vi "headers.vi"(8 "error in (no error)":errorcluster, 10 "string":string, 11 "Byte Stream File in":refnum<file>) -> (0 "error out":errorcluster, 3 "Byte Stream File out":refnum<file>)   [LabVIEW 2019]
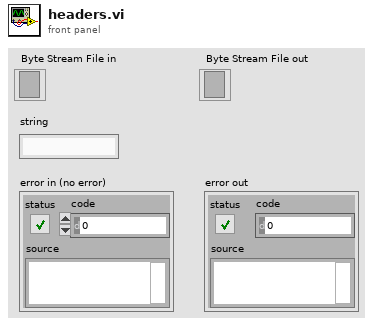
[diagram p1: front panel]
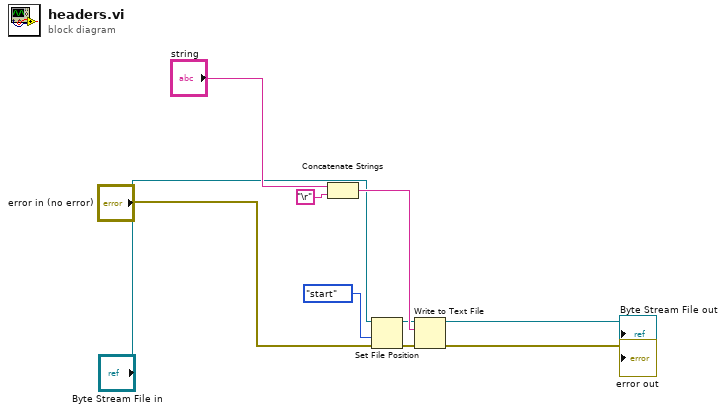
[diagram p0: block diagram]
diagram:
  n1 = Concatenate Strings("string", "\r") -> (w8:string)
  n2 = Set File Position(refnum="Byte Stream File in", from (0:start)=enum16{"start", "end", "current"}."start", error in="error in (no error)") -> (refnum out=w3:refnum<file>, error out=w5:errorcluster)  [unwired: 1 in]
  n3 = Write to Text File(file (use dialog)=w3, text=w8, error in=w5) -> (refnum out=→"Byte Stream File out":refnum<file>, error out=→"error out":errorcluster)  [unwired: 1 in, 1 out]
